vi "Test attach 1.vi"(8 "Error In":errorcluster) -> (0 "Error Out":errorcluster)   [LabVIEW 2014]
uses:
  ServoDatatype.lvclass
panel:
  out "ServoDatatype out":refnum<class "ServoDatatype.lvclass">
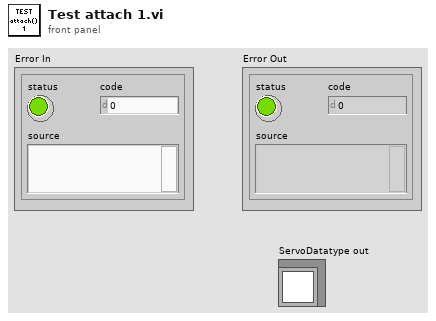
[diagram p1: front panel]
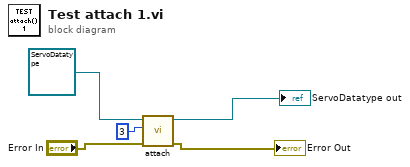
[diagram p0: block diagram]
diagram:
  n1 = call-dynamic "attach.vi"("error in (no error)"="Error In", "pin number"=3, "Servo in"=refnum<class "ServoDatatype.lvclass"> refnum ("ServoDatatype in")) -> ("error out"=→"Error Out":errorcluster, "Servo out"=→"ServoDatatype out":refnum<class "ServoDatatype.lvclass">)  [unwired: 6 in, 1 out]
